vi "Initialize.vi"(8 "error in":errorcluster, 10 "parameters":variant, 11 "PC in":refnum<class "PLTarget PC.lvclass">) -> (0 "error out":errorcluster, 2 "summary":T2[](array[typedef]), 3 "data value reference":T1)   [LabVIEW 2013, in "PLTarget PC.lvclass"]
doc: "This Vi initializes the data of a node its default state.\nThe object is not created inside of this ViI, beacuase it is created from a File depending on user selection."
uses:
  PLTarget PC.lvclass
  <vilib>/NI/Configuration Framework/Node/Summary.ctl
  <vilib>/NI/Configuration Framework/Node/NodeRef.ctl
  <vilib>/NI/Configuration Framework/Node/NISE_CEF_Node.lvclass
  PLTarget PC.lvclass/PLTarget PC.ctl
  <vilib>/NI/Tag Bus Module Framework/root configuration/Target Types.ctl
  Framework Configuration Classes/target configuration/PL_Target Configuration.lvclass/PL_Target Configuration.ctl
  Configuration Editor/Classes/Targets/Targets.lvclass
  <vilib>/NI/Tag Bus Module Framework/root configuration/TBM configuration.lvclass
  Framework Configuration Classes/target configuration/PL_Target Configuration.lvclass
  <vilib>/NI/Configuration Framework/serializable configuration/NISE_CEF_serializable configuration.lvclass
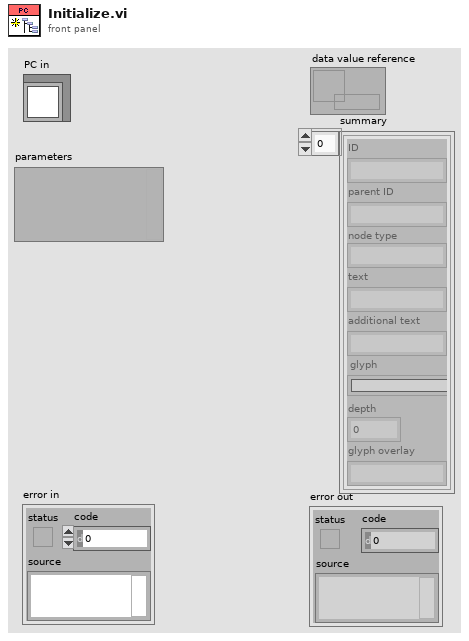
[diagram p1: front panel]
types:
  T1 = typedef "NISE_CEF_Node.lvclass/NodeRef.ctl" = refnum<data-value>
  T2 = typedef "NISE_CEF_Node.lvclass/Summary.ctl" = cluster{"ID":string, "parent ID":string, "node type":string, "text":string, "additional text":string, "glyph":string, "depth":i32, "glyph overlay":string}
  T3 = typedef "TBM configuration.lvclass/Target Types.ctl" = enum16{"Windows", "Mac", "Linux", "Linux RT ARM", "VxWorks", "Pharlap", "Other", "Linux RT x64"}
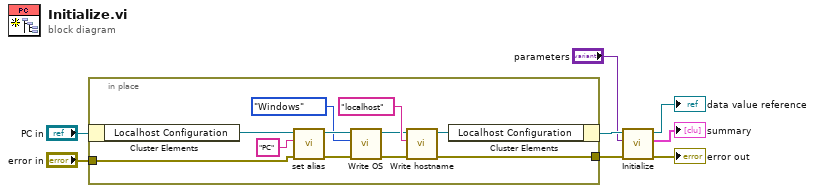
[diagram p0: block diagram]
diagram:
  n1 = in-place {
    in-place-border: "error in" -> [w10]
    in-place-border: [w12] -> w4
    n2 = in-place-cluster #1("PC in") -> ("Localhost Configuration"=w9:refnum<class "PL_Target Configuration.lvclass">)
    n3 = call <vilib>:"set alias.vi"("error in"=w10, "alias"="PC" ("Name"), "configuration in"=w9) -> ("error out"=w13:errorcluster, "configuration out"=w16:refnum<class "PL_Target Configuration.lvclass">)  [unwired: 7 in]
    n4 = call "Write OS.vi"("error in"=w13, "Target Types"=Target_Types."Windows" ("OS"), "PL_Target Configuration in"=w16) -> ("error out"=w18:errorcluster, "PL_Target Configuration out"=w17:refnum<class "PL_Target Configuration.lvclass">)  [unwired: 7 in]
    n5 = call "Write hostname.vi"("error in"=w18, "hostname"="localhost", "PL_Target Configuration in"=w17) -> ("error out"=w12:errorcluster, "PL_Target Configuration out"=w11:refnum<class "PL_Target Configuration.lvclass">)  [unwired: 7 in]
    n6 = in-place-cluster #1("Localhost Configuration"=w11) -> (w5:refnum<class "PLTarget PC.lvclass">)
  }
  n7 = call-parent "Initialize.vi"("error in"=w4, "parameters"="parameters", "node in"=w5) -> ("error out"=→"error out":errorcluster, "summary"=→"summary":T2[], "data value reference"=→"data value reference":T1)  [unwired: 6 in]
